vi "003 abreujatures.vi"() -> ()   [LabVIEW 2019]
panel:
  out "result string":string
  out "element":string
  out "element 2":string
  in  "String":string
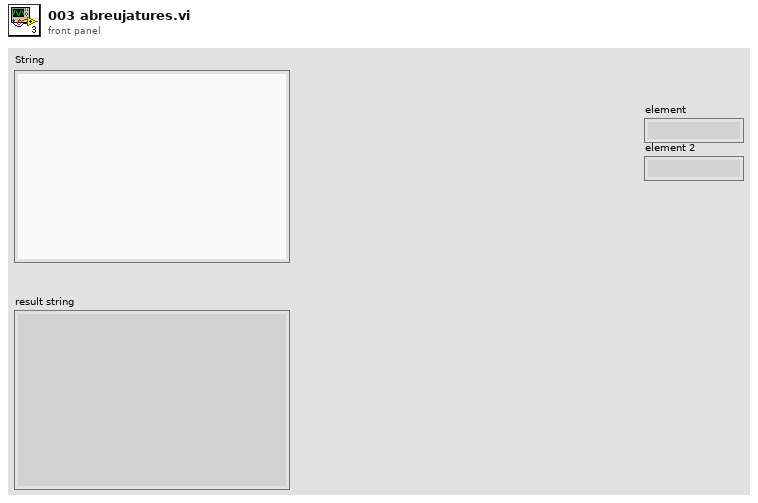
[diagram p1: front panel]
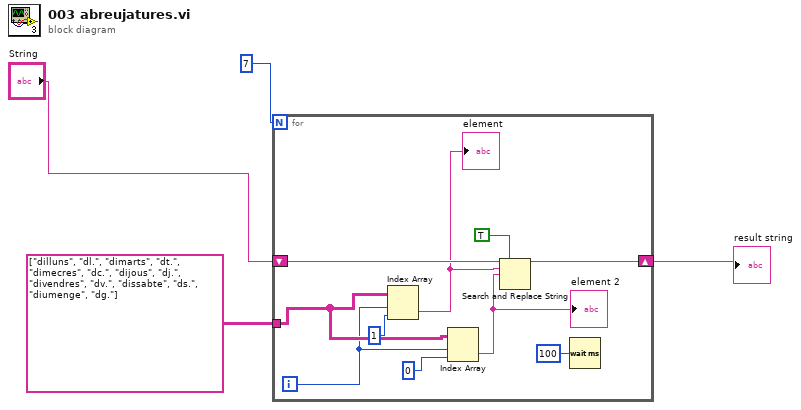
[diagram p0: block diagram]
diagram:
  n1 = for {
    N: 7 -> [_]
    tunnel: string[][] [["dilluns", "dl."], ["dimarts", "dt."], ["dimecres", "dc."], ["dijous", "dj."], ["divendres", "dv."], ["dissabte", "ds."], ["diumenge", "dg."]] -> [w9]
    shift-right: [w12] -> w2
    shift-left: "String" -> [w14]
    i -> [w5]
    n2 = Index Array(array=w9, index (row)=w5, index (col)=1 ("disabled index (col)")) -> (element=w7:string)
    "element" <- w7
    n3 = Index Array(array=w9, index (row)=w5, index (col)=0 ("index (row)")) -> (element=w6:string)
    "element 2" <- w6
    n4 = Search and Replace String(replace all?=TRUE ("replace all? (F)"), input string=w14, search string=w7, replace string=w6) -> (result string=w12:string)  [unwired: 4 in, 3 out]
    n5 = Wait (ms)(milliseconds to wait=u32 100) -> ()  [unwired: 1 out]
  }
  "result string" <- w2
